vi "heartbeat (SubVI).vi"(11 "Denoised Signal":waveform(dbl)) -> (1 "Bradycardia":bool, 2 "Normal":bool, 3 "Tachycardia":bool, 4 "Number of cycles":i32, 5 "Heart Rate":dbl)   [LabVIEW 2024]
uses:
  <vilib>/addons/Biomedical/Biosignal Measurements/Biosignal Preprocessing/subVIs/bmt_Rate Extractor_peak_valley.ctl
  <vilib>/addons/Biomedical/Biosignal Measurements/Biosignal Preprocessing/Biosignal Rate Extractor (Waveform).vi
  <vilib>/addons/Biomedical/NI_BMTK_Measurements.lvlib
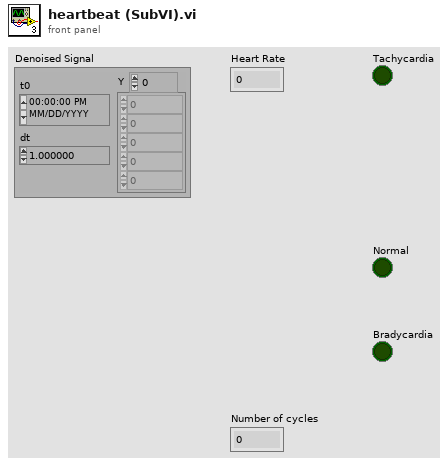
[diagram p1: front panel]
types:
  T1 = typedef "NI_BMTK_Measurements.lvlib/bmt_Rate Extractor_peak_valley.ctl" = u16
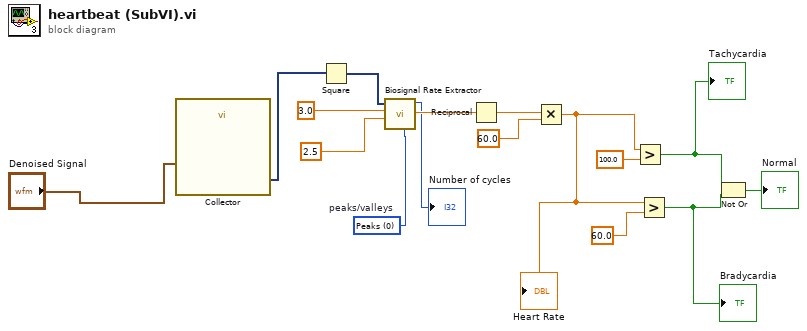
[diagram p0: block diagram]
diagram:
  w16 = T1 0 items=["Peaks", "Valleys"]  # peaks/valleys
  n1 = call "Collector"("Signals"="Denoised Signal") -> ("Collected Signals"=w2:dynamicdata)  [unwired: 9 in, 1 out]
  n2 = Square(x=w2) -> (x^2=w3:dynamicdata)
  n3 = call-poly <vilib>:"Biosignal Rate Extractor.vi"("peaks/valleys"=w16, "low threshold"=2.5, "high threshold"=3.0, "biosignal"=w3) -> ("mean cycle time"=w7:dbl, "number of cycles"=→"Number of cycles":i32)  [unwired: 5 in, 1 out]
  n4 = Reciprocal(x=w7) -> (1/x=w8:dbl)
  n5 = Multiply(x=w8, y=60.0) -> (x*y=w10:dbl)
  "Heart Rate" <- w10
  n6 = Greater?(x=w10, y=100.0) -> (0:w15:bool)
  "Tachycardia" <- w15
  n7 = Greater?(x=w10, y=60.0) -> (0:w14:bool)
  "Bradycardia" <- w14
  n8 = Not Or(1:w14, 2:w15) -> (0:→"Normal":bool)
